vi "SQL_Insert.vi"(6 "columns":string[](array[string]), 7 "create table? (F)":bool, 8 "error in (no error)":errorcluster, 9 "Data":variant, 10 "Table":string, 11 "SQL in":refnum<class "SQL.lvclass">) -> (0 "error out":errorcluster, 3 "SQL out":refnum<class "SQL.lvclass">)   [LabVIEW 2012, in "SQL.lvclass"]
uses:
  SQL.lvclass
  <vilib>/addons/database/NI_Database_API.lvlib
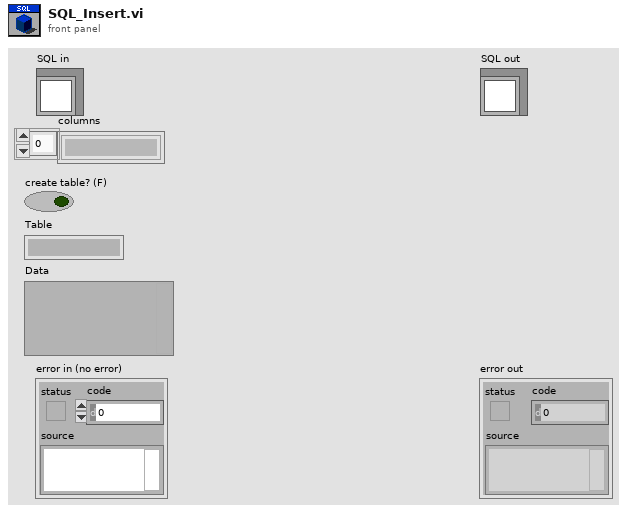
[diagram p1: front panel]
types:
  T1 = typedef "SQL.lvclass/ObjectAttributes.ctl" = cluster{"DB Connection Reference":T2}
  T2 = typedef "NI_Database_API.lvlib/Conn ObjectReference.ctl" = refnum<k1>
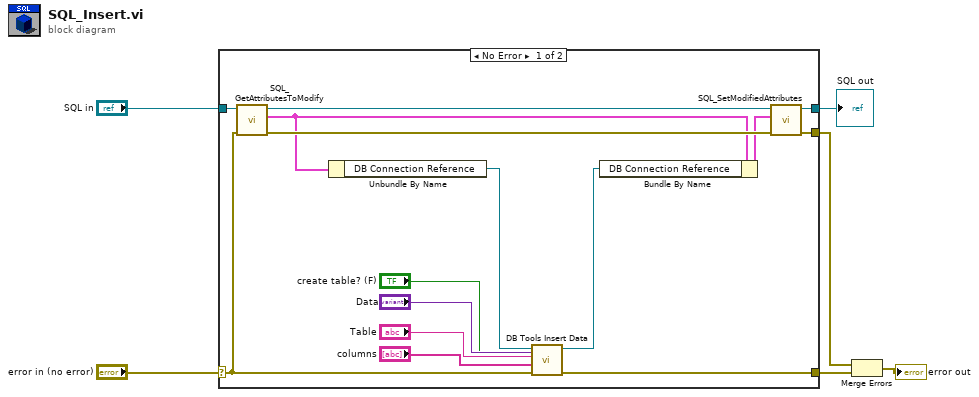
[diagram p0: block diagram]
diagram:
  n1 = case shown="No Error" "error in (no error)" {
    selector: "error in (no error)" -> [w9 w22]
    tunnel: [w21 w22] -> w6
    tunnel: [w16 w23] -> w5
    tunnel: "SQL in" -> [w17 w23]
    tunnel: [w8 w22] -> w1
    frame No Error {
      n2 = call "SQL_GetAttributesToModify.vi"("error in (no error)"=w9, "reference in"=w17) -> ("error out"=w14:errorcluster, "Attributes"=w12:T1, "reference out"=w15:refnum<class "SQL.lvclass">)  [unwired: 6 in, 1 out]
      n3 = Unbundle By Name(w12) -> ("DB Connection Reference"=w11:T2)
      n4 = call <vilib>:"DB Tools Insert Data.vi"("create table? (F)"="create table? (F)", "data"="Data", "error in (no error)"=w9, "columns"="columns", "table"="Table", "connection reference"=w11) -> ("error out"=w21:errorcluster, "connection reference out"=w10:T2)  [unwired: 4 in]
      n5 = Bundle By Name(cluster=w12, "DB Connection Reference"=w10) -> (w13:T1)
      n6 = call "SQL_SetModifiedAttributes.vi"("error in (no error)"=w14, "Attributes"=w13, "reference in"=w15) -> ("error out"=w8:errorcluster, "reference out"=w16:refnum<class "SQL.lvclass">)  [unwired: 7 in]
    }
    frame Error {
    }
  }
  "SQL out" <- w5
  n7 = Merge Errors(w1, w6) -> (→"error out":errorcluster)
